vi "Average(SubVI).vi"(10 "y":dbl, 11 "x":dbl) -> (3 "x/y":dbl)   [LabVIEW 2021]
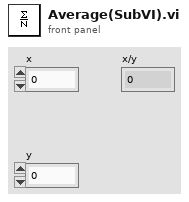
[diagram p1: front panel]
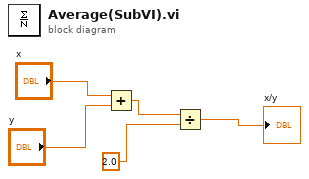
[diagram p0: block diagram]
diagram:
  n1 = Add(x="x", y="y") -> (x+y=w3:dbl)
  n2 = Divide(x=w3, y=2.0) -> (x/y=→"x/y":dbl)
